vi "save images.vi"(0 "Save Folder":string, 1 "File name prefix":string, 2 "Array":T1[](array[typedef]), 3 "error out 2":errorcluster caption="error out", 4 "Bilder/Messschritt":i32) -> (5 "error out":errorcluster)   [LabVIEW 2009]
uses:
  <vilib>/vision/Image Controls.llb/IMAQ Image.ctl
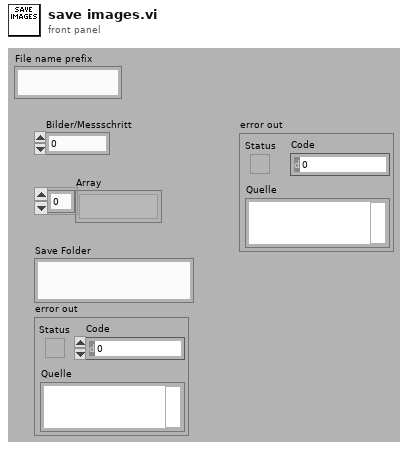
[diagram p1: front panel]
types:
  T1 = typedef "IMAQ Image.ctl" = refnum<image>
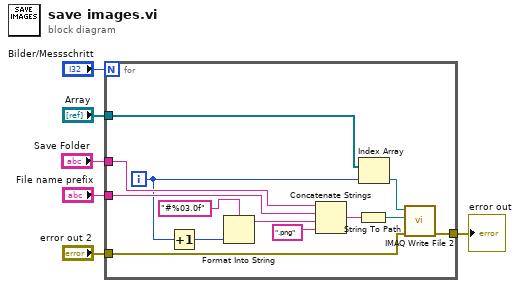
[diagram p0: block diagram]
diagram:
  n1 = for {
    N: "Bilder/Messschritt" -> [_]
    tunnel: "error out 2" -> [w19]
    tunnel: [w18] -> w3
    tunnel: "Save Folder" -> [w15]
    tunnel: "Array" -> [w14]
    tunnel: "File name prefix" -> [w11]
    i -> [w10]
    n2 = Increment(x=w10) -> (x+1=w7:i32)
    n3 = Format Into String(format string="#%03.0f" ("Format-String"), w7) -> (resulting string=w8:string)  [unwired: 2 in, 1 out]
    n4 = Concatenate Strings(w15, w11, w8, ".png" ("String")) -> (w17:string)
    n5 = String To Path(string=w17) -> (path=w16:path)
    n6 = Index Array(array=w14, index=w10) -> (element=w13:T1)
    n7 = call-poly "IMAQ Write File 2"("error in (no error)"=w19, "File Path"=w16, "Image"=w13) -> ("error out"=w18:errorcluster)  [unwired: 7 in, 1 out]
  }
  "error out" <- w3
